vi "routine_ident.vi"(9 "done":dbl, 10 "theta_min":dbl, 11 "theta_max":dbl) -> (3 "routine":dbl)   [LabVIEW 2013]
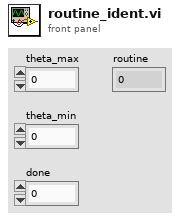
[diagram p1: front panel]
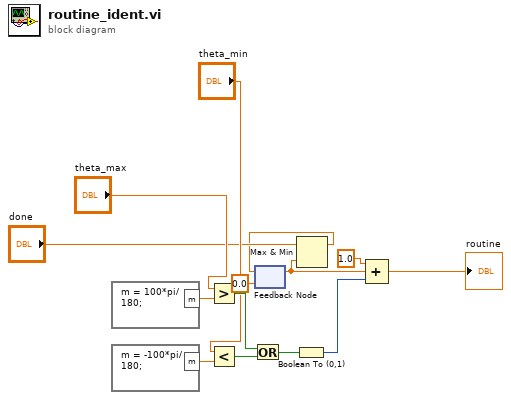
[diagram p0: block diagram]
diagram:
  n1 = formula code="m = 100*pi/180;"() -> ("m"=w6:dbl)
  n2 = formula code="m = -100*pi/180;"() -> ("m"=w8:dbl)
  n3 = Greater?(x="theta_max", y=w6) -> (0:w11:bool)
  n4 = Less?(x="theta_min", y=w8) -> (x < y?=w10:bool)
  n5 = Or(x=w11, y=w10) -> (x .or. y?=w12:bool)
  n6 = feedback #1(0.0) -> (w4:dbl)
  n7 = Boolean To (0,1)(Boolean=w12) -> (0, 1=w13:i16)
  n8 = Max & Min(x="done", y=w4) -> (max(x,y)=w3:dbl)  [unwired: 1 out]
  n9 = feedback-in #1(w3) -> ()
  n10 = Compound Arithmetic op=ADD(1.0 ("value"), w4, w13) -> (→"routine":dbl)
